vi "제목없음 3 (SubVI).vi"(9 "불리언":bool, 10 "문자열 출력 3":string, 11 "문자열":string) -> (3 "문자열 출력 2":string)   [LabVIEW 2018]
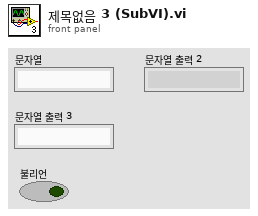
[diagram p1: front panel]
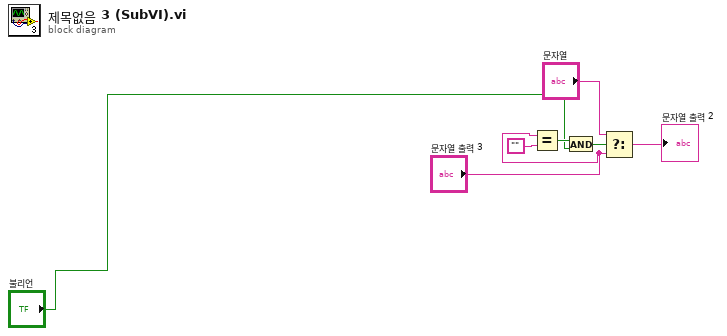
[diagram p0: block diagram]
diagram:
  n1 = Equal?(x="문자열 출력 3", y="") -> (x = y?=w2:bool)
  n2 = And(x=w2, y="불리언") -> (x .and. y?=w3:bool)
  n3 = Select(t="문자열", s=w3, f="문자열 출력 3") -> (s? t:f=→"문자열 출력 2":string)
